vi "Set Class Instance.vi"(11 "Osciloscope Tipe":string) -> (3 "Specific class reference":refnum<class "Tektronic.lvclass">)   [LabVIEW 2020]
uses:
  Class/Tektronic/Tektronic.lvclass
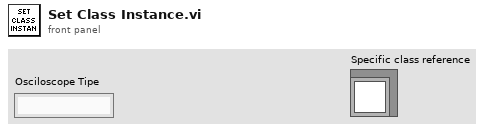
[diagram p1: front panel]
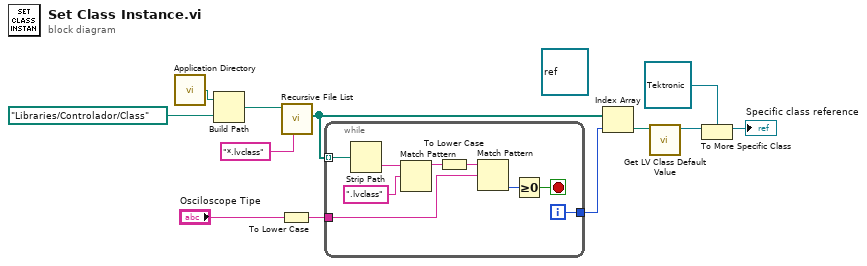
[diagram p0: block diagram]
diagram:
  (unwired) refnum<class> refnum ("LabVIEW Object")
  n1 = call <vilib>:"Application Directory.vi"() -> ("Application Directory"=w11:path)
  n2 = Build Path(base path=w11, name or relative path=path "Libraries/Controlador/Class") -> (appended path=w10:path)
  n3 = To Lower Case(string="Osciloscope Tipe") -> (all lower case string=w7:string)
  n4 = call <vilib>:"Recursive File List.vi"("pattern"="*.lvclass", "Folder Path"=w10) -> ("All Files in Dir"=w6:path[])  [unwired: 5 in, 4 out]
  n5 = while {
    tunnel: w6 -> [w19] mode=indexing
    tunnel: w7 -> [w13]
    tunnel: [w14] -> w5
    i -> [w14]
    stop <- w15 stop-if-true
    n6 = Strip Path(path=w19) -> (name=w20:string)  [unwired: 1 out]
    n7 = Match Pattern(string=w20, regular expression=".lvclass") -> (before substring=w17:string)  [unwired: 1 in, 3 out]
    n8 = To Lower Case(string=w17) -> (all lower case string=w16:string)
    n9 = Match Pattern(string=w16, regular expression=w13) -> (offset past match=w18:i32)  [unwired: 1 in, 3 out]
    n10 = Greater Or Equal To 0?(x=w18) -> (x >= 0?=w15:bool)
  }
  n11 = Index Array(array=w6, index=w5) -> (element=w4:path)
  n12 = call <vilib>:"Get LV Class Default Value.vi"("class path"=w4) -> ("object"=w2:refnum<class>)  [unwired: 9 in, 1 out]
  n13 = To More Specific Class(target class=refnum<class "Tektronic.lvclass"> refnum ("Controlador.lvlib:Tektronic.lvclass"), reference=w2) -> (specific class reference=→"Specific class reference":refnum<class "Tektronic.lvclass">)  [unwired: 1 in, 1 out]
